vi "CA.vi"(0 "init input ports":u8[](array[numeric]), 1 "Alg states":cluster{u32, u8}[](array[cluster]), 5 "output":u8[](array[numeric]), 7 "input ALG msg array":cluster{i32, "Value":string, i32}[](array[cluster]), 9 "Output ALG msg array":cluster{i32, "Value":string, i32}[](array[cluster]), 11 "VOC output msg CASHE":cluster{i32, "Value":string, i32}[](array[cluster]), 12 "ALG output msg CASHE":cluster{i32, "Value":string, i32}[](array[cluster])) -> (3 "Output Alg states":cluster{u32, u8}[](array[cluster]), 4 "input ports":u8[](array[numeric]), 6 "modified output ports":i8[](array[numeric]), 8 "Clear ALG input array":cluster{i32, "Value":string, i32}[](array[cluster]), 10 "Clear ALG output array":cluster{i32, "Value":string, i32}[](array[cluster]), 14 "Curr step msg counter":i32, 15 "Modified ALG output msg CASHE":cluster{i32, "Value":string, i32}[](array[cluster]))   [LabVIEW 2010]
uses:
  bsvt.dll
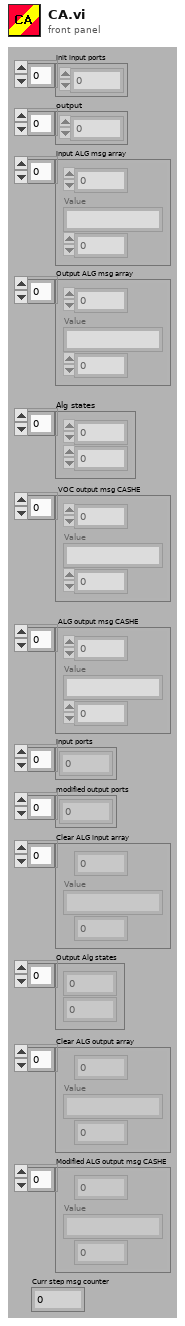
[diagram p1: front panel]
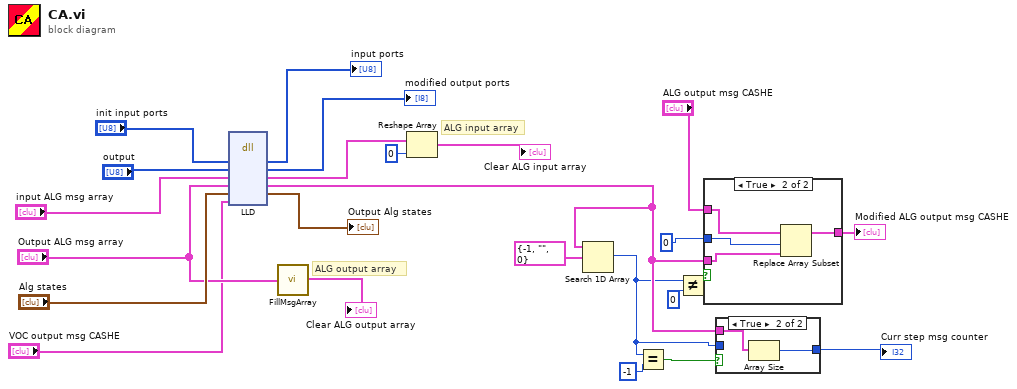
[diagram p0: block diagram]
diagram:
  # "ALG input array"
  # "ALG output array"
  n1 = dll-call lib="D:/Liakh Tanya/Dissertation/Complex/Old BSVT Complex/lib/bsvt.dll" fn="LLD" label="AY"("input"="init input ports", "output"="output", "input ALG msg array"="input ALG msg array", "Output ALG msg array"="Output ALG msg array", "Alg states"="Alg states", "VOC output msg CASHE"="VOC output msg CASHE") -> ("input"=→"input ports":i8[], "output"=→"modified output ports":i8[], "input ALG msg array"=w15:cluster{i32, "Value":string, i32}[], "Output ALG msg array"=w12:cluster{i32, "Value":string, i32}[], "Alg states"=→"Output Alg states":cluster{u32, u8}[])  [unwired: 5 in, 2 out]
  n2 = call "FillMsgArray.vi"("input array"="Output ALG msg array") -> ("output array"=→"Clear ALG output array":cluster{i32, "Value":string, i32}[])
  n3 = Reshape Array(w15, 0 ("dimension size")) -> (→"Clear ALG input array":cluster{i32, "Value":string, i32}[])
  n4 = Search 1D Array(1D array=w12, element=cluster{i32, "Value":string, i32} {-1, "Value"="", 0}) -> (index of element=w11:i32)  [unwired: 1 in]
  n5 = Equal?(x=w11, y=-1) -> (x = y?=w13:bool)
  n6 = Not Equal?(x=w11, y=0) -> (x != y?=w18:bool)
  n7 = case shown="True" w18 {
    tunnel: "ALG output msg CASHE" -> [w25 w26]
    tunnel: 0 -> [_ w28]
    tunnel: w12 -> [_ w29]
    tunnel: [w25 w27] -> w1
    frame False {
    }
    frame True {
      n8 = Replace Array Subset(array=w26, new element=w29, index=w28) -> (w27:cluster{i32, "Value":string, i32}[])
    }
  }
  "Modified ALG output msg CASHE" <- w1
  n9 = case shown="True" w13 {
    tunnel: w12 -> [_ w32]
    tunnel: [w30 w31] -> w10
    tunnel: w11 -> [w30 _]
    frame False {
    }
    frame True {
      n10 = Array Size(array=w32) -> (size(s)=w31:i32)
    }
  }
  "Curr step msg counter" <- w10
